vi "Run all tests.vi"(8 "error in (no error)":errorcluster, 10 "Interactive (T)":bool=TRUE, 11 "Test Report":refnum<class "Test Report.lvclass">) -> (0 "error out":errorcluster, 3 "Test Results":refnum<class "Test Result.lvclass">)   [LabVIEW 2021]
uses:
  <vilib>/addons/_JKI Toolkits/Caraya/classes/Test Result/Test Result.lvclass
  <vilib>/addons/_JKI Toolkits/Caraya/classes/Test Report/Test Report.lvclass
  <vilib>/addons/_JKI Toolkits/Caraya/classes/Test Result/Node Results (Extended).ctl
  <vilib>/addons/_JKI Toolkits/Caraya/classes/Test Result/Test Node (Extended).ctl
  <vilib>/addons/_JKI Toolkits/Caraya/classes/Test Result/Test Registration Data.ctl
  <vilib>/addons/_JKI Toolkits/Caraya/classes/Test Result/Assert Event Data (Extended).ctl
  <vilib>/addons/_JKI Toolkits/Caraya/run-tests/Run Test (Scalar Path).vi
  <vilib>/addons/_JKI Toolkits/Caraya/classes/Test Suite/Test Suite.lvclass
  <vilib>/addons/_JKI Toolkits/Caraya/Caraya.lvlib
panel:
  out "Test Results 2":T1[](array[typedef])
  out "error out 2":errorcluster
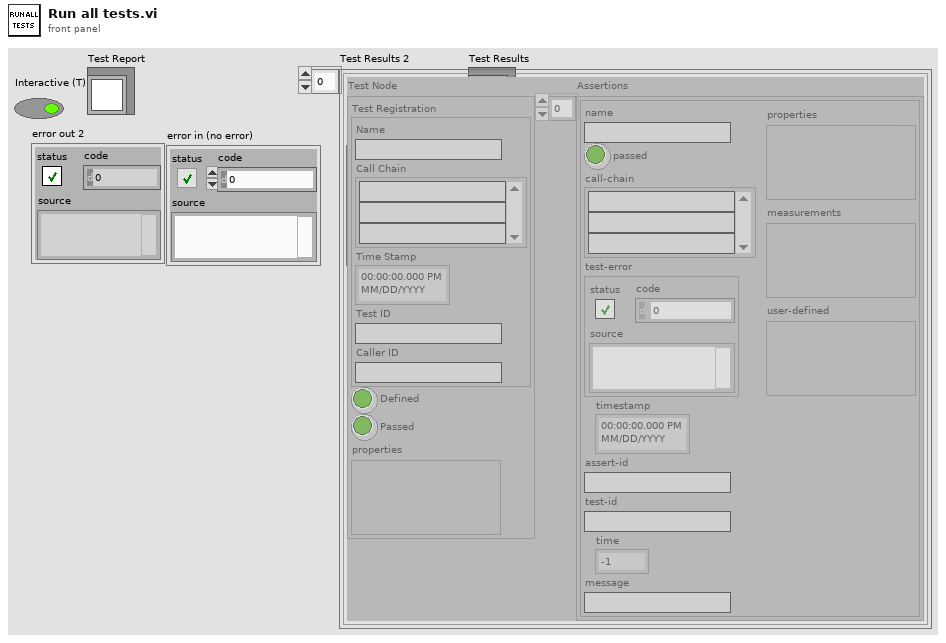
[diagram p1: front panel]
types:
  T1 = typedef "Caraya.lvlib/Test Result.lvclass/Node Results (Extended).ctl" = cluster{"Test Node":T2, "Assertions":T4[]}
  T2 = typedef "Caraya.lvlib/Test Result.lvclass/Test Node (Extended).ctl" = cluster{"Test Registration":T3, "Defined":bool, "Passed":bool, "properties":variant}
  T3 = typedef "Caraya.lvlib/Test Result.lvclass/Test Registration Data.ctl" = cluster{"Name":string, "Call Chain":string[], "Time Stamp":timestamp, "Test ID":string, "Caller ID":string}
  T4 = typedef "Caraya.lvlib/Test Result.lvclass/Assert Event Data (Extended).ctl" = cluster{"name":string, "passed":bool, "call-chain":string[], "test-error":errorcluster, "timestamp":timestamp, "assert-id":string, "test-id":string, "time":dbl, "message":string, "properties":variant, "measurements":variant, "user-defined":variant}
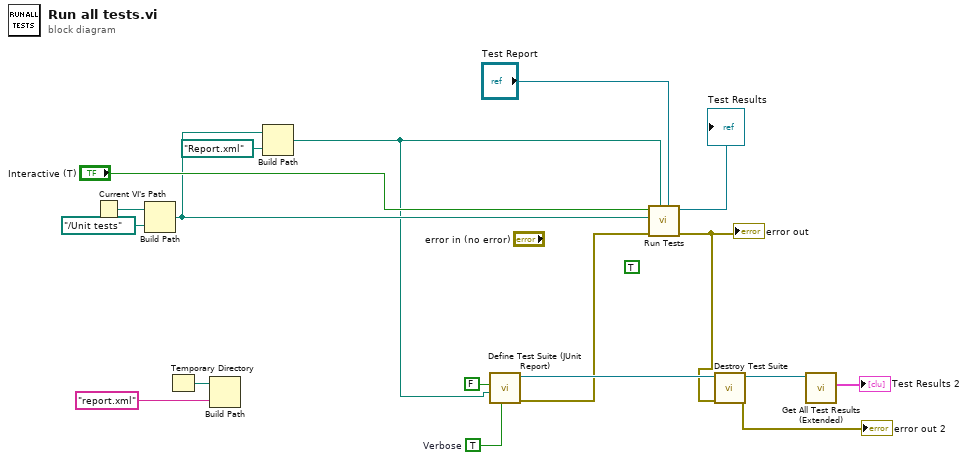
[diagram p0: block diagram]
diagram:
  w5 = TRUE  # Verbose
  (unwired) TRUE ("Verbose")
  n1 = Current VI's Path() -> (path=w18:path)
  n2 = Build Path(base path=w18, name or relative path=path "../Unit tests") -> (appended path=w13:path)
  n3 = Temporary Directory() -> (w11:path)
  n4 = Build Path(base path=w11, name or relative path="report.xml") -> ()  [unwired: 1 out]
  n5 = Build Path(base path=w13, name or relative path=path "Report.xml") -> (appended path=w3:path)
  n6 = call <vilib>:"Define Test Suite (JUnit Report).vi"("Verbose (F)"=w5, "Report Path"=w3, "Interactive"=FALSE) -> ("error out"=w2:errorcluster, "Test Suite"=w6:refnum<class "Test Suite.lvclass">)  [unwired: 6 in, 1 out]
  n7 = call-poly <vilib>:"Run Tests.vi"("Test Report"="Test Report", "Report Path"=w3, "error in"=w2, "Test Path"=w13, "Interactive (T)"="Interactive (T)") -> ("error out"=w1:errorcluster, "Test Results"=→"Test Results":refnum<class "Test Result.lvclass">)  [unwired: 5 in]
  "error out" <- w1
  n8 = call-dynamic "Destroy Test Suite.vi"("error in (no error)"=w1, "Test Suite in"=w6) -> ("error out"=→"error out 2":errorcluster, "Test Suite Results"=w10:refnum<class "Test Result.lvclass">)  [unwired: 8 in]
  n9 = call <vilib>:"Get All Test Results (Extended).vi"("Test Result in"=w10) -> ("Test Results"=→"Test Results 2":T1[])  [unwired: 8 in, 2 out]
